vi "Fn FGV.vi"(7 "Command":T1=enum."Get function", 8 "error in (no error)":errorcluster, 10 "Enum in":T2) -> (0 "error out":errorcluster, 2 "Enum out":T2)   [LabVIEW 2013]
uses:
  Controls/Function States.ctl
  Function Command.ctl
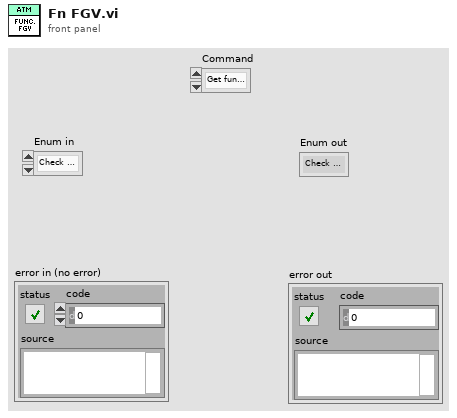
[diagram p1: front panel]
types:
  T1 = typedef "Function Command.ctl" = enum16{"Set function", "Get function"}
  T2 = typedef "Function States.ctl" = enum16{"Check Account", "Deposit", "Withdraw"}
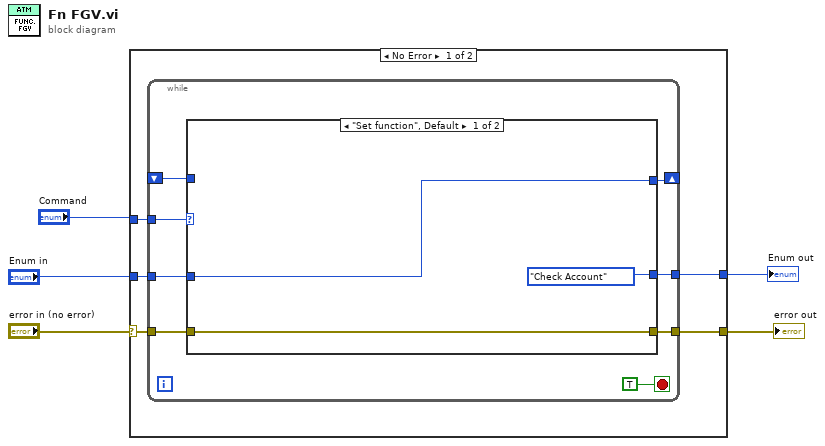
[diagram p0: block diagram]
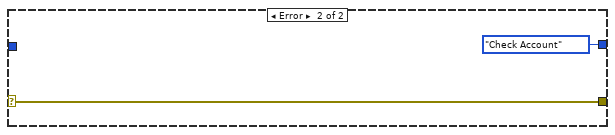
[diagram p3: hidden frame]
diagram:
  n1 = case shown="No Error" "error in (no error)" {
    selector: "error in (no error)" -> [w6 w25]
    tunnel: "Command" -> [w10 _]
    tunnel: "Enum in" -> [w9 _]
    tunnel: [w8 enum16{"Check Account", "Deposit", "Withdraw"}."Check Account" ("Enum")] -> w2
    tunnel: [w7 w25] -> w4
    frame No Error {
      n2 = while {
        tunnel: w10 -> [w18]
        tunnel: w9 -> [w17]
        shift-right: [w16] -> _
        shift-left: _ -> [w15]
        tunnel: [w14] -> w8
        tunnel: w6 -> [w13]
        tunnel: [w12] -> w7
        stop <- TRUE stop-if-true
        n3 = case shown="\"Set function\", Default" w18 {
          tunnel: w17 -> [w21 _]
          tunnel: [w21 w23] -> w16
          tunnel: w15 -> [_ w23]
          tunnel: [Function_States."Check Account" ("Enum in") w23] -> w14
          tunnel: w13 -> [w20 w22]
          tunnel: [w20 w22] -> w12
          frame "Set function", Default {
          }
          frame "Get function" {
          }
        }
      }
    }
    frame Error {
    }
  }
  "error out" <- w4
  "Enum out" <- w2
